vi "Configure Data Format.vi"(0 "VISA resource name":refnum<visa-resource-name>, 5 "Data Format Type (2:Single Precision)":i32(ring)=2 items=["Ascii", "Double-Precision", "Single-Precision"], 11 "error in (no error)":errorcluster) -> (4 "VISA resource name out":refnum<visa-resource-name>, 15 "error out":errorcluster)   [LabVIEW 2020, in "Keithley 2450.lvlib"]
doc: "This sets the data format that is used when transferring readings over the remote interface."
uses:
  <instrlib>/Keithley 2450/Keithley 2450.lvlib
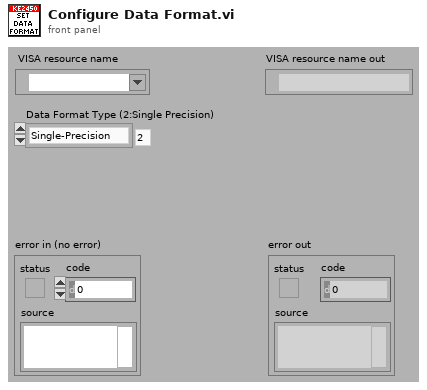
[diagram p1: front panel]
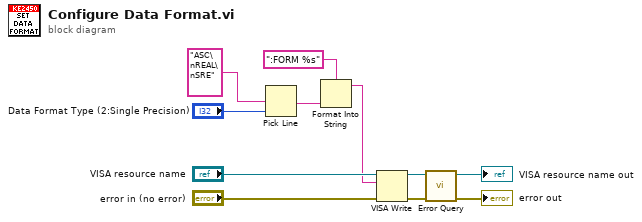
[diagram p0: block diagram]
diagram:
  n1 = Pick Line(multi-line string="ASC\nREAL\nSRE" ("input 1"), line index="Data Format Type (2:Single Precision)") -> (output string=w2:string)  [unwired: 1 in]
  n2 = Format Into String(format string=":FORM %s" ("Fetch Measurement"), w2) -> (resulting string=w5:string)  [unwired: 2 in, 1 out]
  n3 = VISA Write(VISA resource name="VISA resource name", write buffer=w5, error in (no error)="error in (no error)") -> (VISA resource name out=w7:refnum<visa-resource-name>, error out=w6:errorcluster)  [unwired: 1 out]
  n4 = call <instrlib>:"Error Query.vi"("error in (no error)"=w6, "VISA resource name"=w7) -> ("error out"=→"error out":errorcluster, "VISA resource name out"=→"VISA resource name out":refnum<visa-resource-name>)  [unwired: 8 out]
